vi "Scan.vi"(0 "Scan":refnum<vi>, 1 "End":dbl=1.0 format="%.2f", 2 "Start":dbl=1.0 format="%.2f", 3 "Step":dbl=1.0 format="%.2f", 4 "Parameter":variant, 5 "Comment":string, 6 "Unit":string="One", 7 "Prefix":string="Scan-", 8 "Function":string, 9 "Sequencer":string="Sequencer.vi") -> ()   [LabVIEW 2014]
panel:
  in  "data file":refnum<vi>
  in  "Counts":refnum<vi>
  in  "Data":refnum<vi>
  in  "Average Counts or States":refnum<vi>
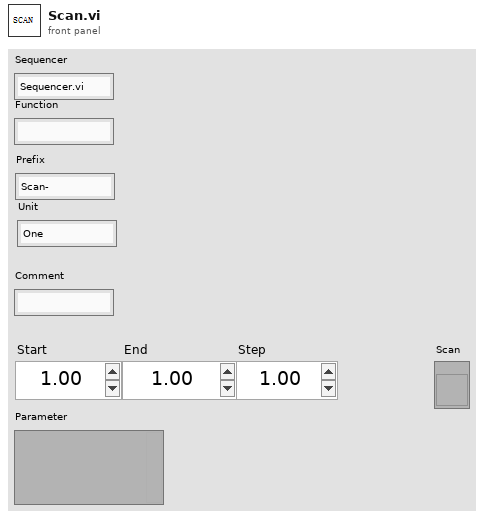
[diagram p1: front panel]
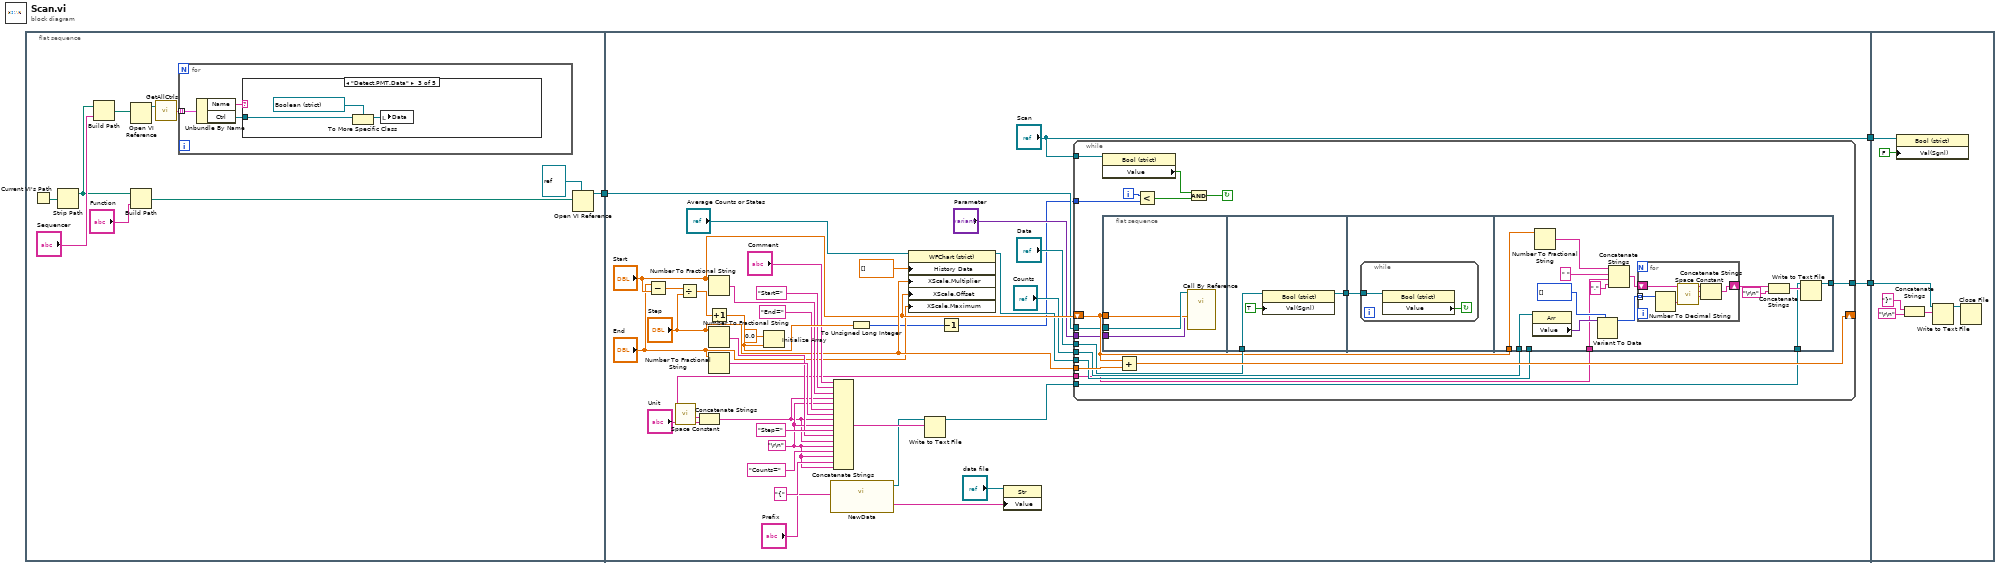
[diagram p0: block diagram]
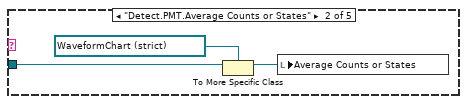
[diagram p3: hidden frame]
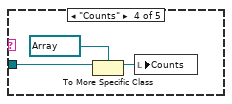
[diagram p4: hidden frame]
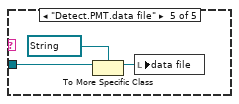
[diagram p5: hidden frame]
diagram:
  n1 = flat-sequence {
    tunnel: [w4] -> w3
    tunnel: w3 -> [w35]
    tunnel: ["Scan"] -> w2
    tunnel: [w30] -> w1
    tunnel: w2 -> [w114]
    tunnel: w1 -> [w113]
    frame #0 {
      n2 = Current VI's Path() -> (path=w13:path)
      n3 = Strip Path(path=w13) -> (stripped path=w6:path)  [unwired: 1 out]
      n4 = Build Path(base path=w6, name or relative path="Sequencer") -> (appended path=w11:path)
      n5 = Open VI Reference(vi path=w11) -> (vi reference=w10:refnum<vi>)  [unwired: 5 in, 1 out]
      n6 = Build Path(base path=w6, name or relative path="Function") -> (appended path=w7:path)
      n7 = call "GetAllCtrls.vi"("VI"=w10) -> ("Ctrls"=w9:cluster{"Name":string, "Ctrl":refnum<vi>}[])  [unwired: 1 in]
      n8 = for {
        tunnel: w9 -> [w16] mode=indexing
        n9 = Unbundle By Name(w16) -> ("Name"=w15:string, "Ctrl"=w14:refnum<vi>)
        n10 = case shown="\"Detect.PMT.Data\"" w15 {
          tunnel: w14 -> [_ w19 w22 w25 w28]
          frame Default {
          }
          frame "Detect.PMT.Average Counts or States" {
            n11 = To More Specific Class(target class=refnum<vi> refnum ("Average Counts or States"), reference=w19) -> (specific class reference=w18:refnum<vi>)  [unwired: 1 in, 1 out]
            n12 = local write "Average Counts or States"(w18) -> ()
          }
          frame "Detect.PMT.Data" {
            n13 = To More Specific Class(target class=refnum<vi> refnum ("Data"), reference=w22) -> (specific class reference=w21:refnum<vi>)  [unwired: 1 in, 1 out]
            n14 = local write "Data"(w21) -> ()
          }
          frame "Counts" {
            n15 = To More Specific Class(target class=refnum<vi> refnum ("Counts"), reference=w25) -> (specific class reference=w24:refnum<vi>)  [unwired: 1 in, 1 out]
            n16 = local write "Counts"(w24) -> ()
          }
          frame "Detect.PMT.data file" {
            n17 = To More Specific Class(target class=refnum<vi> refnum ("data file"), reference=w28) -> (specific class reference=w27:refnum<vi>)  [unwired: 1 in, 1 out]
            n18 = local write "data file"(w27) -> ()
          }
        }
      }
      n19 = Open VI Reference(type specifier VI Refnum (for type only)=refnum<vi> refnum, vi path=w7) -> (vi reference=w4:refnum<vi>)  [unwired: 4 in, 1 out]
    }
    frame #1 {
      w52 = "\r\n"
      n20 = Subtract(x="End", y="Start") -> (x-y=w64:dbl)
      n21 = call <vilib>:"Space Constant.vi"() -> ("String"=w48:string)
      n22 = Divide(x=w64, y="Step") -> (x/y=w63:dbl)
      n23 = Concatenate Strings(w48, "Unit") -> (w49:string)
      n24 = Number To Fractional String(number="Start") -> (F-format string=w59:string)  [unwired: 3 in]
      n25 = Increment(x=w63) -> (x+1=w62:dbl)
      n26 = Number To Fractional String(number="Step") -> (F-format string=w55:string)  [unwired: 3 in]
      n27 = Number To Fractional String(number="End") -> (F-format string=w57:string)  [unwired: 3 in]
      n28 = Initialize Array(0.0 ("element"), w62) -> ()  [unwired: 1 out]
      n29 = call "NewData.vi"("Prefix"="Prefix") -> ("data file name"=w36:string, "data file refnum"=w47:refnum<file>)  [unwired: 2 in]
      n30 = Concatenate Strings("Comment", "Start=" ("string"), w59, w49, w52, "End=" ("string"), w57, w49, w52, "Step=" ("string"), w55, w49, w52, "Counts=" ("string"), w52, "{" ("string"), w52) -> (w60:string)
      n31 = To Unsigned Long Integer(number=w62) -> (unsigned 32bit integer=w32:u32)
      n32 = property class="WFChart (strict)"(reference="Average Counts or States", "History Data"=dbl[] [], "XScale.Multiplier"="Step", "XScale.Offset"="Start", "XScale.Maximum"="End") -> (reference out=w38:refnum<vi>)  [unwired: 1 in, 1 out]
      n33 = Write to Text File(file (use dialog)=w47, text=w60) -> (refnum out=w51:refnum<file>)  [unwired: 2 in, 2 out]
      n34 = Decrement(x=w32) -> (x-1=w29:u32)
      n35 = property class="Str"(reference="data file", "Value"=w36) -> ()  [unwired: 1 in, 2 out]
      n36 = while {
        shift-right: [w83] -> _
        shift-left: "Start" -> [w69]
        tunnel: "Step" -> [w81]
        tunnel: w51 -> [w79]
        tunnel: [w80] -> w30
        tunnel: w29 -> [w76]
        tunnel: "Data" -> [w75]
        tunnel: "Counts" -> [w74]
        tunnel: w38 -> [w72]
        tunnel: "Scan" -> [w70]
        tunnel: w35 -> [w68]
        tunnel: "Parameter" -> [w67]
        tunnel: "Unit" -> [w66]
        i -> [w78]
        stop <- w82 continue-if-true
        n37 = property class="Bool (strict)"(reference=w70) -> ("Value"=w71:bool)  [unwired: 1 in, 2 out]
        n38 = flat-sequence {
          tunnel: w69 -> [w85]
          tunnel: w68 -> [w86]
          tunnel: w67 -> [w84]
          tunnel: w75 -> [w88]
          tunnel: [w87] -> w73
          tunnel: w73 -> [w90]
          tunnel: w69 -> [w105]
          tunnel: w79 -> [w100]
          tunnel: [w99] -> w80
          tunnel: w74 -> [w95]
          tunnel: w72 -> [_]
          tunnel: w66 -> [w94]
          frame #0 {
            n39 = call-by-ref "?"(reference=w86, "Variable"=w85, "Parameter"=w84) -> ()  [unwired: 1 in, 2 out]
          }
          frame #1 {
            n40 = property class="Bool (strict)"(reference=w88, "Val(Sgnl)"=TRUE ("Acquisition")) -> (reference out=w87:refnum<vi>)  [unwired: 1 in, 1 out]
          }
          frame #2 {
            n41 = while {
              tunnel: w90 -> [w92]
              stop <- w91 continue-if-true
              n42 = property class="Bool (strict)"(reference=w92) -> ("Value"=w91:bool)  [unwired: 1 in, 2 out]
            }
          }
          frame #3 {
            n43 = property class="Arr"(reference=w95) -> ("Value"=w98:variant)  [unwired: 1 in, 2 out]
            n44 = Number To Fractional String(number=w105) -> (F-format string=w107:string)  [unwired: 3 in]
            n45 = Variant To Data(type=u32[] [] ("Counts"), Variant=w98) -> (data=w97:u32[])  [unwired: 1 in, 1 out]
            n46 = Concatenate Strings(w107, " " ("string"), w94, "," ("string")) -> (w104:string)
            n47 = for {
              tunnel: w97 -> [w112] mode=indexing
              shift-right: [w110] -> w101
              shift-left: w104 -> [w109]
              n48 = Number To Decimal String(number=w112) -> (decimal integer string=w111:string)  [unwired: 1 in]
              n49 = call <vilib>:"Space Constant.vi"() -> ("String"=w108:string)
              n50 = Concatenate Strings(w109, w108, w111) -> (w110:string)
            }
            n51 = Concatenate Strings(w101, "\r\n") -> (w102:string)
            n52 = Write to Text File(file (use dialog)=w100, text=w102) -> (refnum out=w99:refnum<file>)  [unwired: 2 in, 2 out]
          }
        }
        n53 = Add(x=w69, y=w81) -> (x+y=w83:dbl)
        n54 = Less?(x=w78, y=w76) -> (x < y?=w77:bool)
        n55 = And(x=w71, y=w77) -> (x .and. y?=w82:bool)
      }
    }
    frame #2 {
      n56 = property class="Bool (strict)"(reference=w114, "Val(Sgnl)"=FALSE ("Time Scan")) -> ()  [unwired: 1 in, 2 out]
      n57 = Concatenate Strings("}" ("string"), "\r\n") -> (w115:string)
      n58 = Write to Text File(file (use dialog)=w113, text=w115) -> (refnum out=w118:refnum<file>)  [unwired: 2 in, 2 out]
      n59 = Close File(refnum=w118) -> ()  [unwired: 1 in, 2 out]
    }
  }
